vi "ClusterwitharrayCSG.vi"(1 "Cluster In":cluster{"Array In":csg[], "Numeric Input":csg} {"Numeric Input" format="%.2f"; "Array In" format="%.2f"}, 2 "Base":csg format="%.2f") -> (0 "Cluster Out":cluster{"Array Out":csg[], "Numeric Output":csg} {"Numeric Output" format="%.2f"; "Array Out" format="%.2f"})   [LabVIEW 2011]
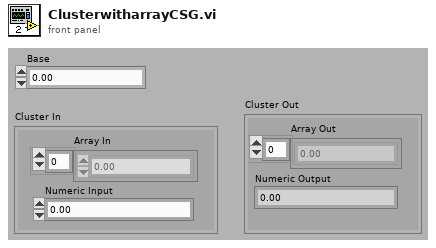
[diagram p1: front panel]
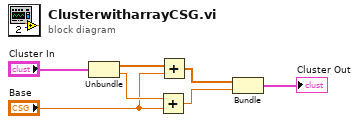
[diagram p0: block diagram]
diagram:
  n1 = Unbundle("Cluster In") -> ("Array In"=w7:csg[], "Numeric Input"=w6:csg)
  n2 = Add(x=w6, y="Base") -> (x+y=w4:csg)
  n3 = Add(x=w7, y="Base") -> (x+y=w5:csg[])
  n4 = Bundle(w5, w4) -> (→"Cluster Out":cluster{csg[], csg})  [unwired: 1 out]
